vi "urscript.vi"(11 "String":string) -> ()   [LabVIEW 2024]
uses:
  <vilib>/RTI DDS Toolkit/Types/RTI DDS Advanced Writer Configuration.ctl
  <vilib>/RTI DDS Toolkit/VIs/AdvancedCreateWriter_String.vi
  <vilib>/RTI DDS Toolkit/VIs/Write_String.vi
  <vilib>/RTI DDS Toolkit/Library/LVDDS_library.lvlib
panel:
  in  "error in (no error)":errorcluster
  in  "Advanced Writer Configuration":T1={"typeName"="std_msgs::msg::dds_::Int32_", "keyName"="", "domainParticipantQoSProfile"="", "dataWriterQoSProfile"="", "forceArrayMapping?"=FALSE, "forceUnboundedString?"=FALSE}
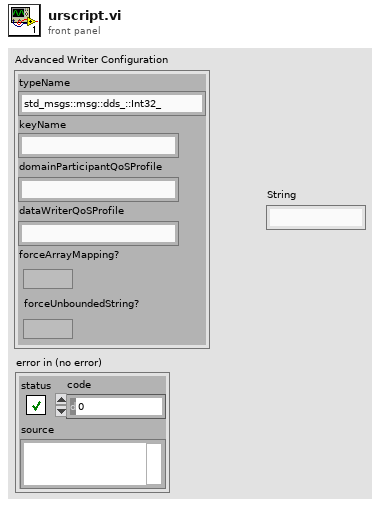
[diagram p1: front panel]
types:
  T1 = typedef "LVDDS_library.lvlib/RTI DDS Advanced Writer Configuration.ctl" = cluster{"typeName":string, "keyName":string, "domainParticipantQoSProfile":string, "dataWriterQoSProfile":string, "forceArrayMapping?":bool, "forceUnboundedString?":bool}
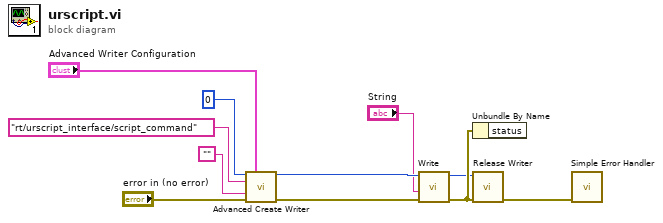
[diagram p0: block diagram]
diagram:
  n1 = call-poly <vilib>:"Advanced Create Writer.vi"("Domain Id"=u32 0, "Advanced Writer Configuration"="Advanced Writer Configuration", "Topic Name"="rt/urscript_interface/script_command", "Data Type"="", "error in (no error)"="error in (no error)") -> ("DDS Object Ref"=w4:u64, "error out"=w5:errorcluster)  [unwired: 9 in]
  n2 = call-poly <vilib>:"Write.vi"("error in (no error)"=w5, "Data"="String", "DDS Object Ref in"=w4) -> ("error out"=w3:errorcluster, "DDS Object Ref out"=w2:u64)  [unwired: 7 in]
  n3 = Unbundle By Name "Unbundle By Name"(w3) -> ()  [unwired: 1 out]
  n4 = call <vilib>:"Release Writer.vi"("error in (no error)"=w3, "DDS Object Ref"=w2) -> ("error out"=w7:errorcluster)  [unwired: 9 in]
  n5 = call <vilib>:"Simple Error Handler.vi"("error in (no error)"=w7) -> ()  [unwired: 4 in, 5 out]
